vi "Get Full Terminal Name_Copy.vi"(8 "error in":errorcluster, 10 "Local Terminal Name":string, 11 "task/channels in":refnum<k21>) -> (0 "error out":errorcluster, 2 "Terminal Name with Device Prefix":tag, 3 "task out":refnum<k21>)   [LabVIEW 2021]
doc: "This example takes in a DAQmx Task and a terminal and converts this to a terminal which includes the device prefix specified in the DAQmx Physical Channel Control.\n\nFor example: \nDAQmx Task/channels in=Dev1/ai1:2\nTerminal=ai/StartTrigger\nDevice+Terminal=/Dev1/ai/StartTrigger"
uses:
  <resource>/objmgr/daqmx.rc
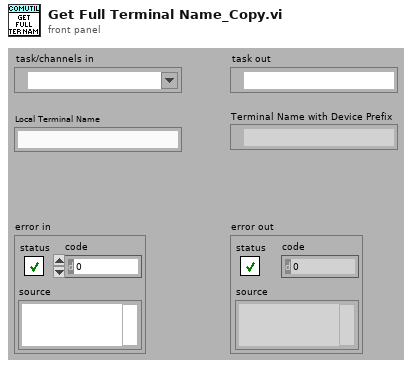
[diagram p1: front panel]
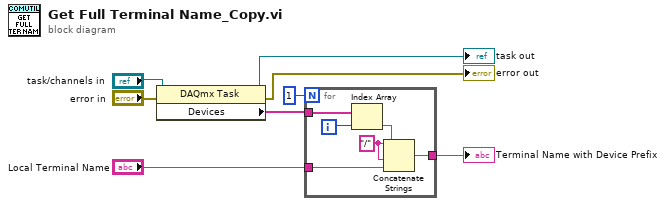
[diagram p0: block diagram]
diagram:
  n1 = property class="DAQmx Task"(reference="task/channels in", error in="error in") -> (reference out=→"task out":refnum<k21>, error out=→"error out":errorcluster, "Devices"=w7:tag[])
  n2 = for {
    N: 1 -> [_]
    tunnel: w7 -> [w14]
    tunnel: "Local Terminal Name" -> [w10]
    tunnel: [w9] -> w4
    i -> [w12]
    w11 = "/" ("string")
    n3 = Index Array(array=w14, index=w12) -> (element=w13:tag)
    n4 = Concatenate Strings(w11, w13, w11, w10) -> (w9:string)
  }
  "Terminal Name with Device Prefix" <- w4
